vi "DefenderPenalty.vi"(6 "N atacantes":u32[](array[numeric]), 10 "Total de n \natacantes":i32, 11 "Robot in":T1={"id"=0, "function"=enum."Attacker", "x"=0.0, "y"=0.0, "orientation"=0.0, "v_tangent"=0.0, "v_normal"=0.0, "v_ang"=0.0, "kick_x"=0.0, "kick_z"=0.0, "dribble"=FALSE, "Timestamp"=timestamp(0 s since 1904-01-01), "dest_x"=0.0, "dest_y"=0.0, "dest_orientation"=0.0, "estimatives"={"est_v_tangent"=0.0, "est_v_normal"=0.0, "est_vx"=0.0, "est_vy"=0.0}, "dest_x_kick"=0.0, "dest_y_kick"=0.0, "Gap Coord"=[], "States"=enum."GoToTangent"}) -> (3 "Robot out":T1={"id"=0, "function"=enum."Attacker", "x"=0.0, "y"=0.0, "orientation"=0.0, "v_tangent"=0.0, "v_normal"=0.0, "v_ang"=0.0, "kick_x"=0.0, "kick_z"=0.0, "dribble"=FALSE, "Timestamp"=timestamp(0 s since 1904-01-01), "dest_x"=0.0, "dest_y"=0.0, "dest_orientation"=0.0, "estimatives"={"est_v_tangent"=0.0, "est_v_normal"=0.0, "est_vx"=0.0, "est_vy"=0.0}, "dest_x_kick"=0.0, "dest_y_kick"=0.0, "Gap Coord"=[], "States"=enum."GoToTangent"})   [LabVIEW 2016]
uses:
  Core/AI Robot.ctl
  Functions Enum.ctl
  AttackerStates.ctl
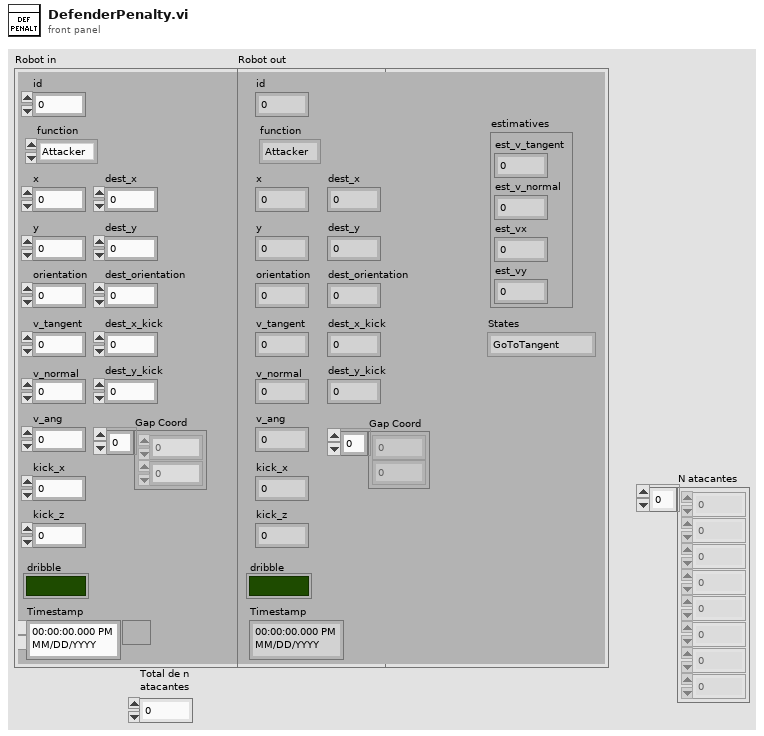
[diagram p1: front panel]
types:
  T1 = typedef "AI Robot.ctl" = cluster{"id":u32, "function":T2, "x":dbl, "y":dbl, "orientation":dbl, "v_tangent":dbl, "v_normal":dbl, "v_ang":dbl, "kick_x":dbl, "kick_z":dbl, "dribble":bool, "Timestamp":timestamp, "dest_x":dbl, "dest_y":dbl, "dest_orientation":dbl, "estimatives":cluster{"est_v_tangent":dbl, "est_v_normal":dbl, "est_vx":dbl, "est_vy":dbl}, "dest_x_kick":dbl, "dest_y_kick":dbl, "Gap Coord":dbl[], "States":T3}
  T2 = typedef "Functions Enum.ctl" = enum16{"Attacker", "Goalie", "Defender", "Striker", "Goto 0", "Dummy", "Kicker", "ZigZag"}
  T3 = typedef "AttackerStates.ctl" = enum16{"Pass", "GoToTangent", "BallGetting", "GoToKick", ""}
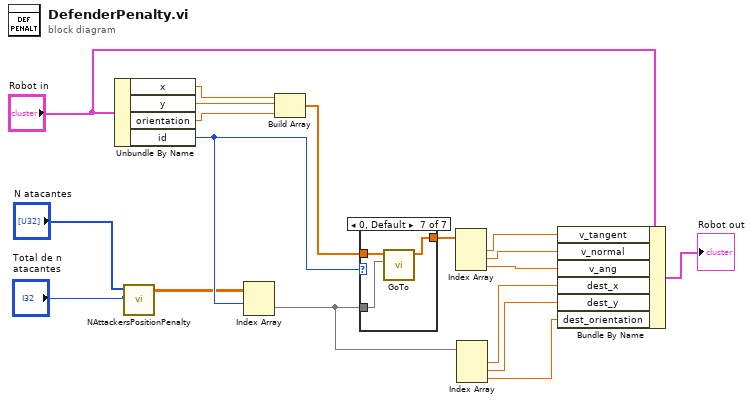
[diagram p0: block diagram]
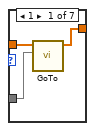
[diagram p2: hidden frame]
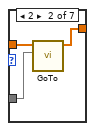
[diagram p3: hidden frame]
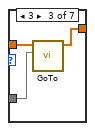
[diagram p4: hidden frame]
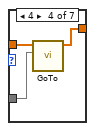
[diagram p5: hidden frame]
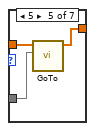
[diagram p6: hidden frame]
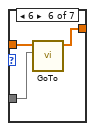
[diagram p7: hidden frame]
diagram:
  n1 = Unbundle By Name("Robot in") -> ("x"=w18:dbl, "y"=w17:dbl, "orientation"=w16:dbl, "id"=w8:u32)
  n2 = call "NAttackersPositionPenalty.vi"("N atacantes"="N atacantes", "Total de n \natacantes"="Total de n \natacantes") -> ("Posição dos não atacantes\ndurante o penalte"=w7:dbl[][])  [unwired: 8 in]
  n3 = Index Array(array=w7, index (row)=w8) -> (element=w4:dbl[])  [unwired: 1 in]
  n4 = Build Array(w18, w17, w16) -> (w15:dbl[])
  n5 = case shown="0, Default" w8 {
    tunnel: w15 -> [w21 w24 w27 w30 w33 w36 w39]
    tunnel: [w20 w23 w26 w29 w32 w35 w38] -> w14
    tunnel: w4 -> [w19 w22 w25 w28 w31 w34 w37]
    frame 1 {
      n6 = call "GoTo.vi"("Target"=w19, "Position"=w21) -> ("Output\nVelocity"=w20:dbl[])  [unwired: 8 in, 1 out]
    }
    frame 2 {
      n7 = call "GoTo.vi"("Target"=w22, "Position"=w24) -> ("Output\nVelocity"=w23:dbl[])  [unwired: 8 in, 1 out]
    }
    frame 3 {
      n8 = call "GoTo.vi"("Target"=w25, "Position"=w27) -> ("Output\nVelocity"=w26:dbl[])  [unwired: 8 in, 1 out]
    }
    frame 4 {
      n9 = call "GoTo.vi"("Target"=w28, "Position"=w30) -> ("Output\nVelocity"=w29:dbl[])  [unwired: 8 in, 1 out]
    }
    frame 5 {
      n10 = call "GoTo.vi"("Target"=w31, "Position"=w33) -> ("Output\nVelocity"=w32:dbl[])  [unwired: 8 in, 1 out]
    }
    frame 6 {
      n11 = call "GoTo.vi"("Target"=w34, "Position"=w36) -> ("Output\nVelocity"=w35:dbl[])  [unwired: 8 in, 1 out]
    }
    frame 0, Default {
      n12 = call "GoTo.vi"("Target"=w37, "Position"=w39) -> ("Output\nVelocity"=w38:dbl[])  [unwired: 8 in, 1 out]
    }
  }
  n13 = Index Array(array=w14) -> (element #1=w12:dbl, element #2=w11:dbl, element #3=w10:dbl)  [unwired: 3 in]
  n14 = Index Array(array=w4) -> (element #1=w3:dbl, element #2=w2:dbl, element #3=w1:dbl)  [unwired: 3 in]
  n15 = Bundle By Name(cluster="Robot in", "v_tangent"=w12, "v_normal"=w11, "v_ang"=w10, "dest_x"=w3, "dest_y"=w2, "dest_orientation"=w1) -> (→"Robot out":T1)
